vi "Comments.Create Lockin Filter Description.vi"(7 "error in (no error)":errorcluster, 10 "Control Experiment":refnum<class "Control Experiment.lvclass">) -> (0 "error out":errorcluster, 2 "Filter Section":string, 3 "Control Experiment out":refnum<class "Control Experiment.lvclass">)   [LabVIEW 2016, in "Control Experiment.lvclass"]
uses:
  Control Experiment.lvclass
  Control Experiment.lvclass/Control Experiment.ctl
  <userlib>/LevyLab/Lockin-Multichannel/Instrument.Lockin/Instrument.Lockin.lvclass
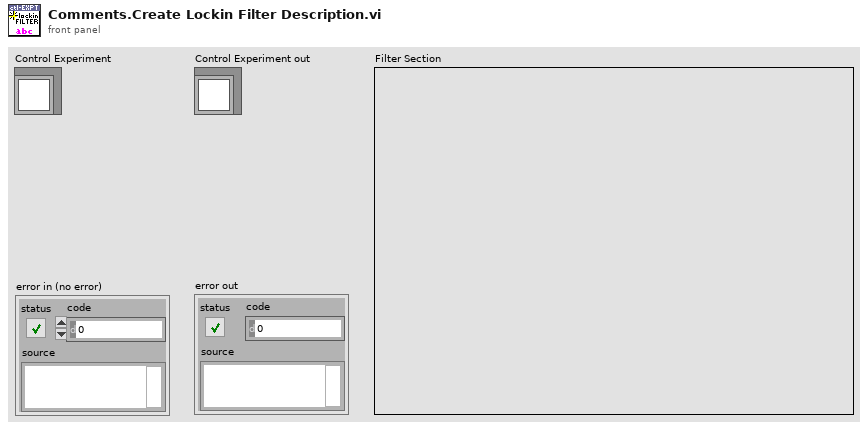
[diagram p1: front panel]
types:
  T1 = typedef "Instrument.Lockin.lvclass/REF filter-cluster.ctl" = cluster{"TC (s)":dbl, "order":i32}
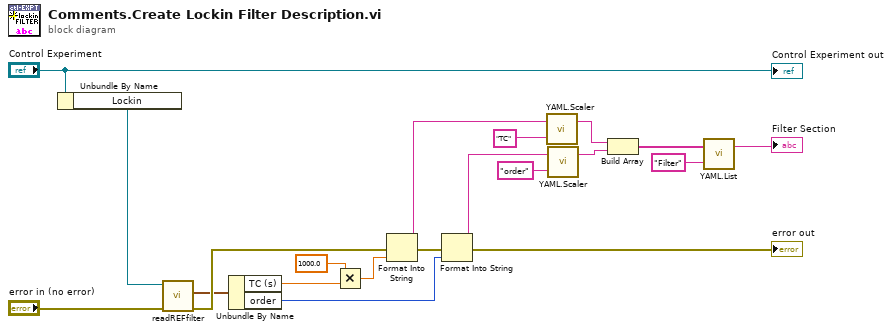
[diagram p0: block diagram]
diagram:
  n1 = Unbundle By Name("Control Experiment") -> ("Lockin"=w2:refnum<class "Instrument.Lockin.lvclass">)
  n2 = call <userlib>:"readREFfilter.vi"("error in (no error)"="error in (no error)", "Instrument.Lockin in"=w2) -> ("error out"=w14:errorcluster, "REF filter"=w5:T1)  [unwired: 7 in, 1 out]
  n3 = Unbundle By Name(w5) -> ("TC (s)"=w18:dbl, "order"=w3:i32)
  n4 = Multiply(x=1000.0, y=w18) -> (x*y=w17:dbl)
  n5 = Format Into String(error in=w14, w17) -> (resulting string=w11:string, error out=w20:errorcluster)  [unwired: 2 in]
  n6 = Format Into String(error in=w20, w3) -> (resulting string=w12:string, error out=→"error out":errorcluster)  [unwired: 2 in]
  n7 = call "YAML.Scaler.vi"("Key"="TC", "Scaler"=w11) -> ("Output"=w9:string)  [unwired: 1 in]
  n8 = call "YAML.Scaler.vi"("Key"="order", "Scaler"=w12) -> ("Output"=w8:string)  [unwired: 1 in]
  n9 = Build Array(w9, w8) -> (w4:string[])
  n10 = call "YAML.List.vi"("Key"="Filter" ("string"), "lines"=w4) -> ("Output"=→"Filter Section":string)  [unwired: 1 in]
  "Control Experiment out" <- "Control Experiment"
